vi "Excel Packing & Format.vi"(0 "Settings Cluster":T1={"Supply Voltage [Vdc]"=14.4, "Max Supply Current [Idc]"=50.0, "Settling Delay"=0.0, "Temp Criteria"=0.0, "Voltage Steps [Vrms]"=[0.0, 0.25, 0.5, 1.0, 1.95, 3.0, 3.9, 5.5], "User Notes"="", "Config Wave File Path"=path "", "Config Voltage [Vrms]"=0.1, "Channel Configuration List"={"Channel Configuration Cluster"={"Input"=enum."1 AVG", "Enable"=FALSE, "User Notes"="", "Voltage Range"=15.0, "Current Range"=2.5}, "Channel Configuration Cluster 2"={"Input"=enum."1", "Enable"=FALSE, "User Notes"="", "Voltage Range"=15.0, "Current Range"=2.5}, "Channel Configuration Cluster 3"={"Input"=enum."1", "Enable"=FALSE, "User Notes"="", "Voltage Range"=15.0, "Current Range"=2.5}, "Channel Configuration Cluster 4"={"Input"=enum."1", "Enable"=FALSE, "User Notes"="", "Voltage Range"=15.0, "Current Range"=2.5}, "Channel Configuration Cluster 5"={"Input"=enum."1", "Enable"=FALSE, "User Notes"="", "Voltage Range"=15.0, "Current Range"=2.5}, "Channel Configuration Cluster 6"={"Input"=enum."1", "Enable"=FALSE, "User Notes"="", "Voltage Range"=15.0, "Current Range"=2.5}, "Channel Configuration Cluster 7"={"Input"=enum."1", "Enable"=FALSE, "User Notes"="", "Voltage Range"=15.0, "Current Range"=2.5}, "Channel Configuration Cluster 8"={"Input"=enum."1", "Enable"=FALSE, "User Notes"="", "Voltage Range"=15.0, "Current Range"=2.5}, "Channel Configuration Cluster 9"={"Input"=enum."1", "Enable"=FALSE, "User Notes"="", "Voltage Range"=15.0, "Current Range"=2.5}, "Channel Configuration Cluster 10"={"Input"=enum."1", "Enable"=FALSE, "User Notes"="", "Voltage Range"=15.0, "Current Range"=25.0}, "Channel Configuration Cluster 11"={"Input"=enum."1", "Enable"=FALSE, "User Notes"="", "Voltage Range"=15.0, "Current Range"=25.0}, "Channel Configuration Cluster 12"={"Input"=enum."1", "Enable"=FALSE, "User Notes"="", "Voltage Range"=15.0, "Current Range"=25.0}, "Channel Configuration Cluster 13"={"Input"=enum."1", "Enable"=FALSE, "User Notes"="", "Voltage Range"=15.0, "Current Range"=25.0}, "Channel Configuration Cluster 14"={"Input"=enum."1", "Enable"=FALSE, "User Notes"="", "Voltage Range"=15.0, "Current Range"=25.0}, "Channel Configuration Cluster 15"={"Input"=enum."1", "Enable"=FALSE, "User Notes"="", "Voltage Range"=15.0, "Current Range"=25.0}, "Channel Configuration Cluster 16"={"Input"=enum."1", "Enable"=FALSE, "User Notes"="", "Voltage Range"=15.0, "Current Range"=25.0}, "Channel Configuration Cluster 17"={"Input"=enum."1", "Enable"=FALSE, "User Notes"="", "Voltage Range"=15.0, "Current Range"=25.0}}, "User Gains"={"Gain 1"=0.0, "Gain 2"=0.0, "Gain 3"=0.0, "Gain 4"=0.0, "Gain 5"=0.0, "Gain 6"=0.0}, "Gains"={"Gain 1"=0.0, "Gain 2"=0.0, "Gain 3"=0.0, "Gain 4"=0.0, "Gain 5"=0.0, "Gain 6"=0.0}, "Gain Array"={"Gain 1"=0.0, "Gain 2"=0.0, "Gain 3"=0.0, "Gain 4"=0.0, "Gain 5"=0.0, "Gain 6"=0.0, "Gain 7"=0.0, "Gain 8"=0.0, "Gain 9"=0.0, "Gain 10"=0.0, "Gain 11"=0.0, "Gain 12"=0.0, "Gain 13"=0.0, "Gain 14"=0.0, "Gain 15"=0.0, "Gain 16"=0.0, "Gain 17"=0.0}, "Wave File Path 1"=path "", "Wave File Path 2"=path "", "Wave File Path 3"=path "", "Wave File Path 4"=path "", "Range"=FALSE, "CF"=FALSE} {"Gain Array"."Gain 17" format="%.2f"; "Gain Array"."Gain 16" format="%.2f"; "Gain Array"."Gain 15" format="%.2f"; "Gain Array"."Gain 14" format="%.2f"; "Gain Array"."Gain 13" format="%.2f"; "Gain Array"."Gain 12" format="%.2f"; "Gain Array"."Gain 11" format="%.2f"; "Gain Array"."Gain 10" format="%.2f"; "Gain Array"."Gain 9" format="%.2f"; "Gain Array"."Gain 8" format="%.2f"; "Gain Array"."Gain 7" format="%.2f"; "Gain Array"."Gain 6" format="%.2f"; "Gain Array"."Gain 5" format="%.2f"; "Gain Array"."Gain 4" format="%.2f"; "Gain Array"."Gain 3" format="%.2f"; "Gain Array"."Gain 2" format="%.2f"; "Gain Array"."Gain 1" format="%.2f"; "Gains"."Gain 6" format="%.2f"; "Gains"."Gain 5" format="%.2f"; "Gains"."Gain 4" format="%.2f"; "Gains"."Gain 3" format="%.2f"; "Gains"."Gain 2" format="%.2f"; "Gains"."Gain 1" format="%.2f"; "User Gains"."Gain 6" format="%.2f"; "User Gains"."Gain 5" format="%.2f"; "User Gains"."Gain 4" format="%.2f"; "User Gains"."Gain 3" format="%.2f"; "User Gains"."Gain 2" format="%.2f"; "User Gains"."Gain 1" format="%.2f"; "Channel Configuration List"."Channel Configuration Cluster 17"."Current Range" items=["1 <500m>"=0.5, "2 <1>"=1.0, "5 <2.5>"=2.5, "10 <5>"=5.0, "20 <10>"=10.0, "50 <25>"=25.0]; "Channel Configuration List"."Channel Configuration Cluster 17"."Voltage Range" items=["1.5 <0.75>"=0.75, "3 <1.5>"=1.5, "6 <3>"=3.0, "10 <5>"=5.0, "15 <7.5>"=7.5, "30 <15>"=15.0, "60 <30>"=30.0, "100 <50>"=50.0, "150 <75>"=75.0, "300 <150>"=150.0, "600 <300>"=300.0, "1000 <500>"=500.0]; "Channel Configuration List"."Channel Configuration Cluster 16"."Current Range" items=["1 <500m>"=0.5, "2 <1>"=1.0, "5 <2.5>"=2.5, "10 <5>"=5.0, "20 <10>"=10.0, "50 <25>"=25.0]; "Channel Configuration List"."Channel Configuration Cluster 16"."Voltage Range" items=["1.5 <0.75>"=0.75, "3 <1.5>"=1.5, "6 <3>"=3.0, "10 <5>"=5.0, "15 <7.5>"=7.5, "30 <15>"=15.0, "60 <30>"=30.0, "100 <50>"=50.0, "150 <75>"=75.0, "300 <150>"=150.0, "600 <300>"=300.0, "1000 <500>"=500.0]; "Channel Configuration List"."Channel Configuration Cluster 15"."Current Range" items=["1 <500m>"=0.5, "2 <1>"=1.0, "5 <2.5>"=2.5, "10 <5>"=5.0, "20 <10>"=10.0, "50 <25>"=25.0]; "Channel Configuration List"."Channel Configuration Cluster 15"."Voltage Range" items=["1.5 <0.75>"=0.75, "3 <1.5>"=1.5, "6 <3>"=3.0, "10 <5>"=5.0, "15 <7.5>"=7.5, "30 <15>"=15.0, "60 <30>"=30.0, "100 <50>"=50.0, "150 <75>"=75.0, "300 <150>"=150.0, "600 <300>"=300.0, "1000 <500>"=500.0]; "Channel Configuration List"."Channel Configuration Cluster 14"."Current Range" items=["1 <500m>"=0.5, "2 <1>"=1.0, "5 <2.5>"=2.5, "10 <5>"=5.0, "20 <10>"=10.0, "50 <25>"=25.0]; "Channel Configuration List"."Channel Configuration Cluster 14"."Voltage Range" items=["1.5 <0.75>"=0.75, "3 <1.5>"=1.5, "6 <3>"=3.0, "10 <5>"=5.0, "15 <7.5>"=7.5, "30 <15>"=15.0, "60 <30>"=30.0, "100 <50>"=50.0, "150 <75>"=75.0, "300 <150>"=150.0, "600 <300>"=300.0, "1000 <500>"=500.0]; "Channel Configuration List"."Channel Configuration Cluster 13"."Current Range" items=["1 <500m>"=0.5, "2 <1>"=1.0, "5 <2.5>"=2.5, "10 <5>"=5.0, "20 <10>"=10.0, "50 <25>"=25.0]; "Channel Configuration List"."Channel Configuration Cluster 13"."Voltage Range" items=["1.5 <0.75>"=0.75, "3 <1.5>"=1.5, "6 <3>"=3.0, "10 <5>"=5.0, "15 <7.5>"=7.5, "30 <15>"=15.0, "60 <30>"=30.0, "100 <50>"=50.0, "150 <75>"=75.0, "300 <150>"=150.0, "600 <300>"=300.0, "1000 <500>"=500.0]; "Channel Configuration List"."Channel Configuration Cluster 12"."Current Range" items=["1 <500m>"=0.5, "2 <1>"=1.0, "5 <2.5>"=2.5, "10 <5>"=5.0, "20 <10>"=10.0, "50 <25>"=25.0]; "Channel Configuration List"."Channel Configuration Cluster 12"."Voltage Range" items=["1.5 <0.75>"=0.75, "3 <1.5>"=1.5, "6 <3>"=3.0, "10 <5>"=5.0, "15 <7.5>"=7.5, "30 <15>"=15.0, "60 <30>"=30.0, "100 <50>"=50.0, "150 <75>"=75.0, "300 <150>"=150.0, "600 <300>"=300.0, "1000 <500>"=500.0]; "Channel Configuration List"."Channel Configuration Cluster 11"."Current Range" items=["1 <500m>"=0.5, "2 <1>"=1.0, "5 <2.5>"=2.5, "10 <5>"=5.0, "20 <10>"=10.0, "50 <25>"=25.0]; "Channel Configuration List"."Channel Configuration Cluster 11"."Voltage Range" items=["1.5 <0.75>"=0.75, "3 <1.5>"=1.5, "6 <3>"=3.0, "10 <5>"=5.0, "15 <7.5>"=7.5, "30 <15>"=15.0, "60 <30>"=30.0, "100 <50>"=50.0, "150 <75>"=75.0, "300 <150>"=150.0, "600 <300>"=300.0, "1000 <500>"=500.0]; "Channel Configuration List"."Channel Configuration Cluster 10"."Current Range" items=["1 <500m>"=0.5, "2 <1>"=1.0, "5 <2.5>"=2.5, "10 <5>"=5.0, "20 <10>"=10.0, "50 <25>"=25.0]; "Channel Configuration List"."Channel Configuration Cluster 10"."Voltage Range" items=["1.5 <0.75>"=0.75, "3 <1.5>"=1.5, "6 <3>"=3.0, "10 <5>"=5.0, "15 <7.5>"=7.5, "30 <15>"=15.0, "60 <30>"=30.0, "100 <50>"=50.0, "150 <75>"=75.0, "300 <150>"=150.0, "600 <300>"=300.0, "1000 <500>"=500.0]; "Channel Configuration List"."Channel Configuration Cluster 9"."Voltage Range" items=["1.5 <0.75>"=0.75, "3 <1.5>"=1.5, "6 <3>"=3.0, "10 <5>"=5.0, "15 <7.5>"=7.5, "30 <15>"=15.0, "60 <30>"=30.0, "100 <50>"=50.0, "150 <75>"=75.0, "300 <150>"=150.0, "600 <300>"=300.0, "1000 <500>"=500.0]; "Channel Configuration List"."Channel Configuration Cluster 9"."Current Range" items=["10m <5m>"=0.005, "20m <10m>"=0.01, "50m <25m>"=0.025, "100m <50m>"=0.05, "200m <100m>"=0.1, "500m <250m>"=0.25, "1 <500m>"=0.5, "2 <1>"=1.0, "5 <2.5>"=2.5]; "Channel Configuration List"."Channel Configuration Cluster 8"."Voltage Range" items=["1.5 <0.75>"=0.75, "3 <1.5>"=1.5, "6 <3>"=3.0, "10 <5>"=5.0, "15 <7.5>"=7.5, "30 <15>"=15.0, "60 <30>"=30.0, "100 <50>"=50.0, "150 <75>"=75.0, "300 <150>"=150.0, "600 <300>"=300.0, "1000 <500>"=500.0]; "Channel Configuration List"."Channel Configuration Cluster 8"."Current Range" items=["10m <5m>"=0.005, "20m <10m>"=0.01, "50m <25m>"=0.025, "100m <50m>"=0.05, "200m <100m>"=0.1, "500m <250m>"=0.25, "1 <500m>"=0.5, "2 <1>"=1.0, "5 <2.5>"=2.5]; "Channel Configuration List"."Channel Configuration Cluster 7"."Voltage Range" items=["1.5 <0.75>"=0.75, "3 <1.5>"=1.5, "6 <3>"=3.0, "10 <5>"=5.0, "15 <7.5>"=7.5, "30 <15>"=15.0, "60 <30>"=30.0, "100 <50>"=50.0, "150 <75>"=75.0, "300 <150>"=150.0, "600 <300>"=300.0, "1000 <500>"=500.0]; "Channel Configuration List"."Channel Configuration Cluster 7"."Current Range" items=["10m <5m>"=0.005, "20m <10m>"=0.01, "50m <25m>"=0.025, "100m <50m>"=0.05, "200m <100m>"=0.1, "500m <250m>"=0.25, "1 <500m>"=0.5, "2 <1>"=1.0, "5 <2.5>"=2.5]; "Channel Configuration List"."Channel Configuration Cluster 6"."Voltage Range" items=["1.5 <0.75>"=0.75, "3 <1.5>"=1.5, "6 <3>"=3.0, "10 <5>"=5.0, "15 <7.5>"=7.5, "30 <15>"=15.0, "60 <30>"=30.0, "100 <50>"=50.0, "150 <75>"=75.0, "300 <150>"=150.0, "600 <300>"=300.0, "1000 <500>"=500.0]; "Channel Configuration List"."Channel Configuration Cluster 6"."Current Range" items=["10m <5m>"=0.005, "20m <10m>"=0.01, "50m <25m>"=0.025, "100m <50m>"=0.05, "200m <100m>"=0.1, "500m <250m>"=0.25, "1 <500m>"=0.5, "2 <1>"=1.0, "5 <2.5>"=2.5]; "Channel Configuration List"."Channel Configuration Cluster 5"."Voltage Range" items=["1.5 <0.75>"=0.75, "3 <1.5>"=1.5, "6 <3>"=3.0, "10 <5>"=5.0, "15 <7.5>"=7.5, "30 <15>"=15.0, "60 <30>"=30.0, "100 <50>"=50.0, "150 <75>"=75.0, "300 <150>"=150.0, "600 <300>"=300.0, "1000 <500>"=500.0]; "Channel Configuration List"."Channel Configuration Cluster 5"."Current Range" items=["10m <5m>"=0.005, "20m <10m>"=0.01, "50m <25m>"=0.025, "100m <50m>"=0.05, "200m <100m>"=0.1, "500m <250m>"=0.25, "1 <500m>"=0.5, "2 <1>"=1.0, "5 <2.5>"=2.5]; "Channel Configuration List"."Channel Configuration Cluster 4"."Voltage Range" items=["1.5 <0.75>"=0.75, "3 <1.5>"=1.5, "6 <3>"=3.0, "10 <5>"=5.0, "15 <7.5>"=7.5, "30 <15>"=15.0, "60 <30>"=30.0, "100 <50>"=50.0, "150 <75>"=75.0, "300 <150>"=150.0, "600 <300>"=300.0, "1000 <500>"=500.0]; "Channel Configuration List"."Channel Configuration Cluster 4"."Current Range" items=["10m <5m>"=0.005, "20m <10m>"=0.01, "50m <25m>"=0.025, "100m <50m>"=0.05, "200m <100m>"=0.1, "500m <250m>"=0.25, "1 <500m>"=0.5, "2 <1>"=1.0, "5 <2.5>"=2.5]; "Channel Configuration List"."Channel Configuration Cluster 3"."Voltage Range" items=["1.5 <0.75>"=0.75, "3 <1.5>"=1.5, "6 <3>"=3.0, "10 <5>"=5.0, "15 <7.5>"=7.5, "30 <15>"=15.0, "60 <30>"=30.0, "100 <50>"=50.0, "150 <75>"=75.0, "300 <150>"=150.0, "600 <300>"=300.0, "1000 <500>"=500.0]; "Channel Configuration List"."Channel Configuration Cluster 3"."Current Range" items=["10m <5m>"=0.005, "20m <10m>"=0.01, "50m <25m>"=0.025, "100m <50m>"=0.05, "200m <100m>"=0.1, "500m <250m>"=0.25, "1 <500m>"=0.5, "2 <1>"=1.0, "5 <2.5>"=2.5]; "Channel Configuration List"."Channel Configuration Cluster 2"."Voltage Range" items=["1.5 <0.75>"=0.75, "3 <1.5>"=1.5, "6 <3>"=3.0, "10 <5>"=5.0, "15 <7.5>"=7.5, "30 <15>"=15.0, "60 <30>"=30.0, "100 <50>"=50.0, "150 <75>"=75.0, "300 <150>"=150.0, "600 <300>"=300.0, "1000 <500>"=500.0]; "Channel Configuration List"."Channel Configuration Cluster 2"."Current Range" items=["10m <5m>"=0.005, "20m <10m>"=0.01, "50m <25m>"=0.025, "100m <50m>"=0.05, "200m <100m>"=0.1, "500m <250m>"=0.25, "1 <500m>"=0.5, "2 <1>"=1.0, "5 <2.5>"=2.5]; "Channel Configuration List"."Channel Configuration Cluster"."Voltage Range" items=["1.5 <0.75>"=0.75, "3 <1.5>"=1.5, "6 <3>"=3.0, "10 <5>"=5.0, "15 <7.5>"=7.5, "30 <15>"=15.0, "60 <30>"=30.0, "100 <50>"=50.0, "150 <75>"=75.0, "300 <150>"=150.0, "600 <300>"=300.0, "1000 <500>"=500.0]; "Channel Configuration List"."Channel Configuration Cluster"."Current Range" items=["10m <5m>"=0.005, "20m <10m>"=0.01, "50m <25m>"=0.025, "100m <50m>"=0.05, "200m <100m>"=0.1, "500m <250m>"=0.25, "1 <500m>"=0.5, "2 <1>"=1.0, "5 <2.5>"=2.5]; "Settling Delay" min=0.0 format="%<%H:%M:%S>t"}, 1 "Datalog Cluster Array":T7[](array[typedef]) {"WT1800 Averages"."Vrms" format="%.3f"; "WT1800 Averages"."Irms" format="%.3f"; "WT1800 Averages"."Power" format="%.3f"; "WT1800 Averages"."Vpkpk" format="%.3f"; "WT1800 Averages"."Ipkpk" format="%.3f"; "WT1800 Measurements"."Vrms" format="%.3f"; "WT1800 Measurements"."Irms" format="%.3f"; "WT1800 Measurements"."Power" format="%.3f"; "WT1800 Measurements"."Vpkpk" format="%.3f"; "WT1800 Measurements"."Ipkpk" format="%.3f"; "DSA Averages"."Vrms" format="%.3f"; "DSA Averages"."Vdc" format="%.3f"; "DSA Averages"."Vpk+" format="%.3f"; "DSA Averages"."Vpk-" format="%.3f"; "DSA Averages"."Vpkpk" format="%.3f"; "DSA Measurements"."Vrms" format="%.3f"; "DSA Measurements"."Vdc" format="%.3f"; "DSA Measurements"."Vpk+" format="%.3f"; "DSA Measurements"."Vpk-" format="%.3f"; "DSA Measurements"."Vpkpk" format="%.3f"}) -> (7 "Irms":dbl[][](array[numeric]), 8 "Heat":dbl[](array[numeric]), 9 "Power":dbl[][](array[numeric]), 10 "DSA Averages":T13[][](array[typedef]) {"Vrms" format="%.3f"; "Vdc" format="%.3f"; "Vpk+" format="%.3f"; "Vpk-" format="%.3f"; "Vpkpk" format="%.3f"}, 11 "Vrms":dbl[][](array[numeric]), 12 "Enable CH":bool[](array[boolean]), 13 "Vpp":dbl[][](array[numeric]), 14 "Voltage Steps [Vrms]":dbl[](array[numeric]), 15 "Voltage Step":string[](array[string]), 16 "CH#":string[](array[string]), 17 "Ipp":dbl[][](array[numeric]), 18 "WT1800 Averages":T10[][](array[typedef]) {"Vrms" format="%.3f"; "Irms" format="%.3f"; "Power" format="%.3f"; "Vpkpk" format="%.3f"; "Ipkpk" format="%.3f"}, 19 "Cluster":T14)   [LabVIEW 2015]
uses:
  Controls/DSA Readings.ctl
  Controls/WT1800 Readings.ctl
  Controls/Datalog Bundle Control.ctl
  Controls/WT1800 Functions.ctl
  Controls/WT1800 Measurements.ctl
  Controls/DSA Functions.ctl
  Controls/DSA Measurements.ctl
  Controls/Settings Control.ctl
  Controls/Channel Configuration List.ctl
  Controls/Channel Configuration Cluster.ctl
  Controls/Channel Configuration Cluster High Current.ctl
  Controls/Gain Averages.ctl
  Controls/Gain Array.ctl
panel:
  out "NICH1_Vrms":string[](array[string])
  out "NICH2_Vrms":string[](array[string])
  out "NICH2_Vpp":string[](array[string])
  out "NICH1_Vpp":string[](array[string])
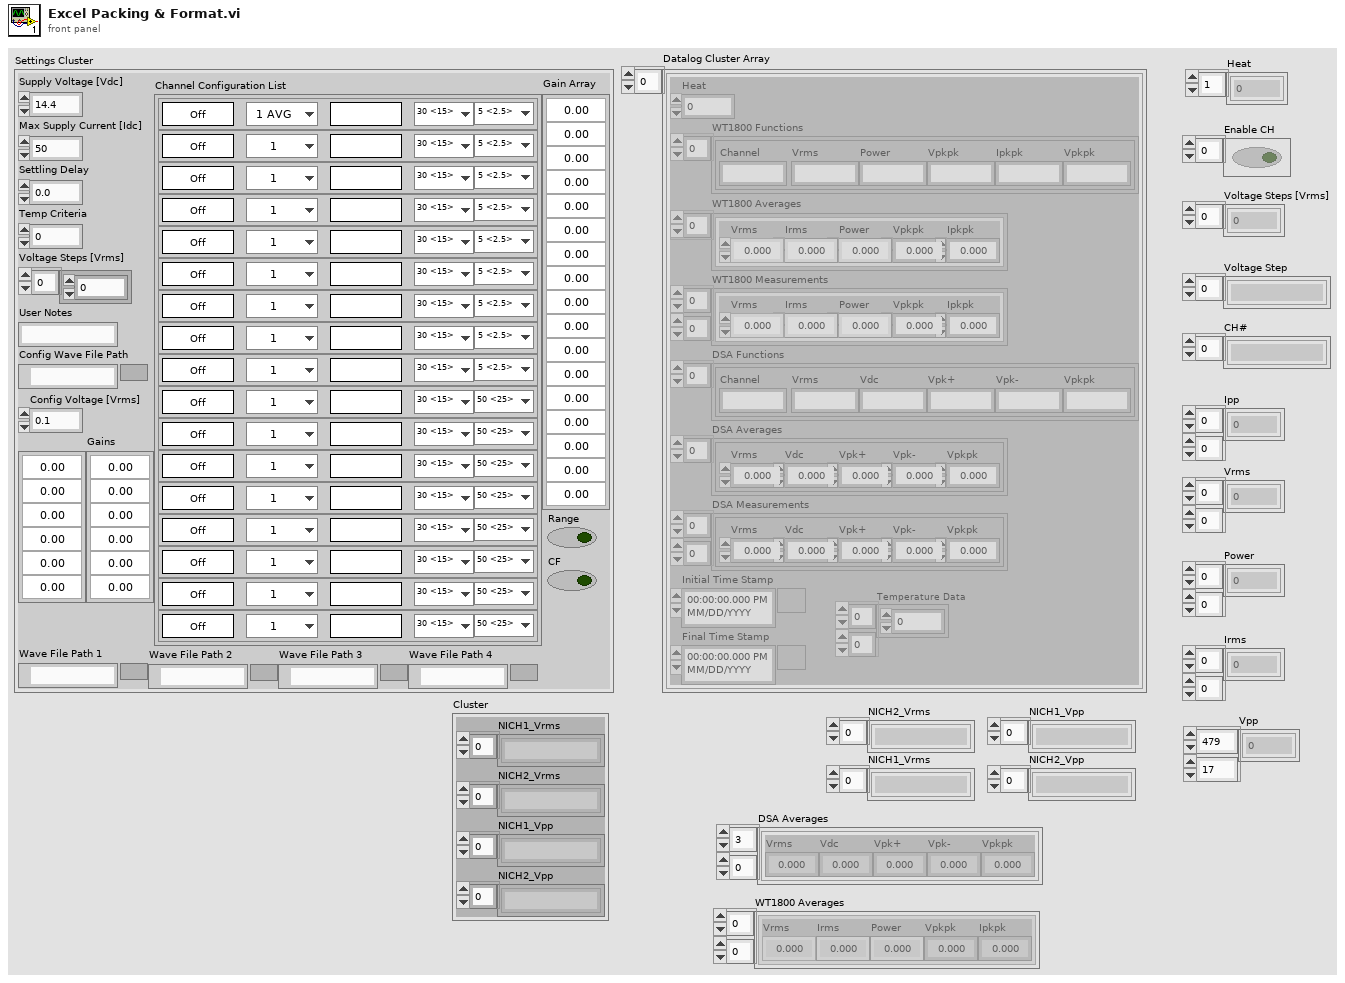
[diagram p1: front panel]
types:
  T1 = typedef "Settings Control.ctl" = cluster{"Supply Voltage [Vdc]":dbl, "Max Supply Current [Idc]":dbl, "Settling Delay":dbl, "Temp Criteria":dbl, "Voltage Steps [Vrms]":dbl[], "User Notes":string, "Config Wave File Path":path, "Config Voltage [Vrms]":dbl, "Channel Configuration List":T2, "User Gains":T5, "Gains":T5, "Gain Array":T6, "Wave File Path 1":path, "Wave File Path 2":path, "Wave File Path 3":path, "Wave File Path 4":path, "Range":bool, "CF":bool}
  T2 = typedef "Channel Configuration List.ctl" = cluster{"Channel Configuration Cluster":T3, "Channel Configuration Cluster 2":T3, "Channel Configuration Cluster 3":T3, "Channel Configuration Cluster 4":T3, "Channel Configuration Cluster 5":T3, "Channel Configuration Cluster 6":T3, "Channel Configuration Cluster 7":T3, "Channel Configuration Cluster 8":T3, "Channel Configuration Cluster 9":T3, "Channel Configuration Cluster 10":T4, "Channel Configuration Cluster 11":T4, "Channel Configuration Cluster 12":T4, "Channel Configuration Cluster 13":T4, "Channel Configuration Cluster 14":T4, "Channel Configuration Cluster 15":T4, "Channel Configuration Cluster 16":T4, "Channel Configuration Cluster 17":T4}
  T3 = typedef "Channel Configuration Cluster.ctl" = cluster{"Input":enum16{"---", "1", "1 AVG", "2", "2 AVG", "3", "3 AVG", "4", "4 AVG"}, "Enable":bool, "User Notes":string, "Voltage Range":dbl, "Current Range":dbl}
  T4 = typedef "Channel Configuration Cluster High Current.ctl" = cluster{"Input":enum16{"---", "1", "1 AVG", "2", "2 AVG", "3", "3 AVG", "4", "4 AVG"}, "Enable":bool, "User Notes":string, "Voltage Range":dbl, "Current Range":dbl}
  T5 = typedef "Gain Averages.ctl" = cluster{"Gain 1":dbl, "Gain 2":dbl, "Gain 3":dbl, "Gain 4":dbl, "Gain 5":dbl, "Gain 6":dbl}
  T6 = typedef "Gain Array.ctl" = cluster{"Gain 1":dbl, "Gain 2":dbl, "Gain 3":dbl, "Gain 4":dbl, "Gain 5":dbl, "Gain 6":dbl, "Gain 7":dbl, "Gain 8":dbl, "Gain 9":dbl, "Gain 10":dbl, "Gain 11":dbl, "Gain 12":dbl, "Gain 13":dbl, "Gain 14":dbl, "Gain 15":dbl, "Gain 16":dbl, "Gain 17":dbl}
  T7 = typedef "Datalog Bundle Control.ctl" = cluster{"Heat":dbl, "WT1800 Functions":T8, "WT1800 Averages":T9, "WT1800 Measurements":T10[][], "DSA Functions":T11, "DSA Averages":T12, "DSA Measurements":T13[][], "Initial Time Stamp":timestamp, "Final Time Stamp":timestamp, "Temperature Data":dbl[][]}
  T8 = typedef "WT1800 Functions.ctl" = cluster{"Channel":string, "Vrms":string, "Power":string, "Vpkpk":string, "Ipkpk":string, "Vpkpk":string}[]
  T9 = typedef "WT1800 Measurements.ctl" = T10[]
  T10 = typedef "WT1800 Readings.ctl" = cluster{"Vrms":dbl, "Irms":dbl, "Power":dbl, "Vpkpk":dbl, "Ipkpk":dbl}
  T11 = typedef "DSA Functions.ctl" = cluster{"Channel":string, "Vrms":string, "Vdc":string, "Vpk+":string, "Vpk-":string, "Vpkpk":string}[]
  T12 = typedef "DSA Measurements.ctl" = T13[]
  T13 = typedef "DSA Readings.ctl" = cluster{"Vrms":dbl, "Vdc":dbl, "Vpk+":dbl, "Vpk-":dbl, "Vpkpk":dbl}
  T14 = cluster{"NICH1_Vrms":string[], "NICH2_Vrms":string[], "NICH1_Vpp":string[], "NICH2_Vpp":string[]}
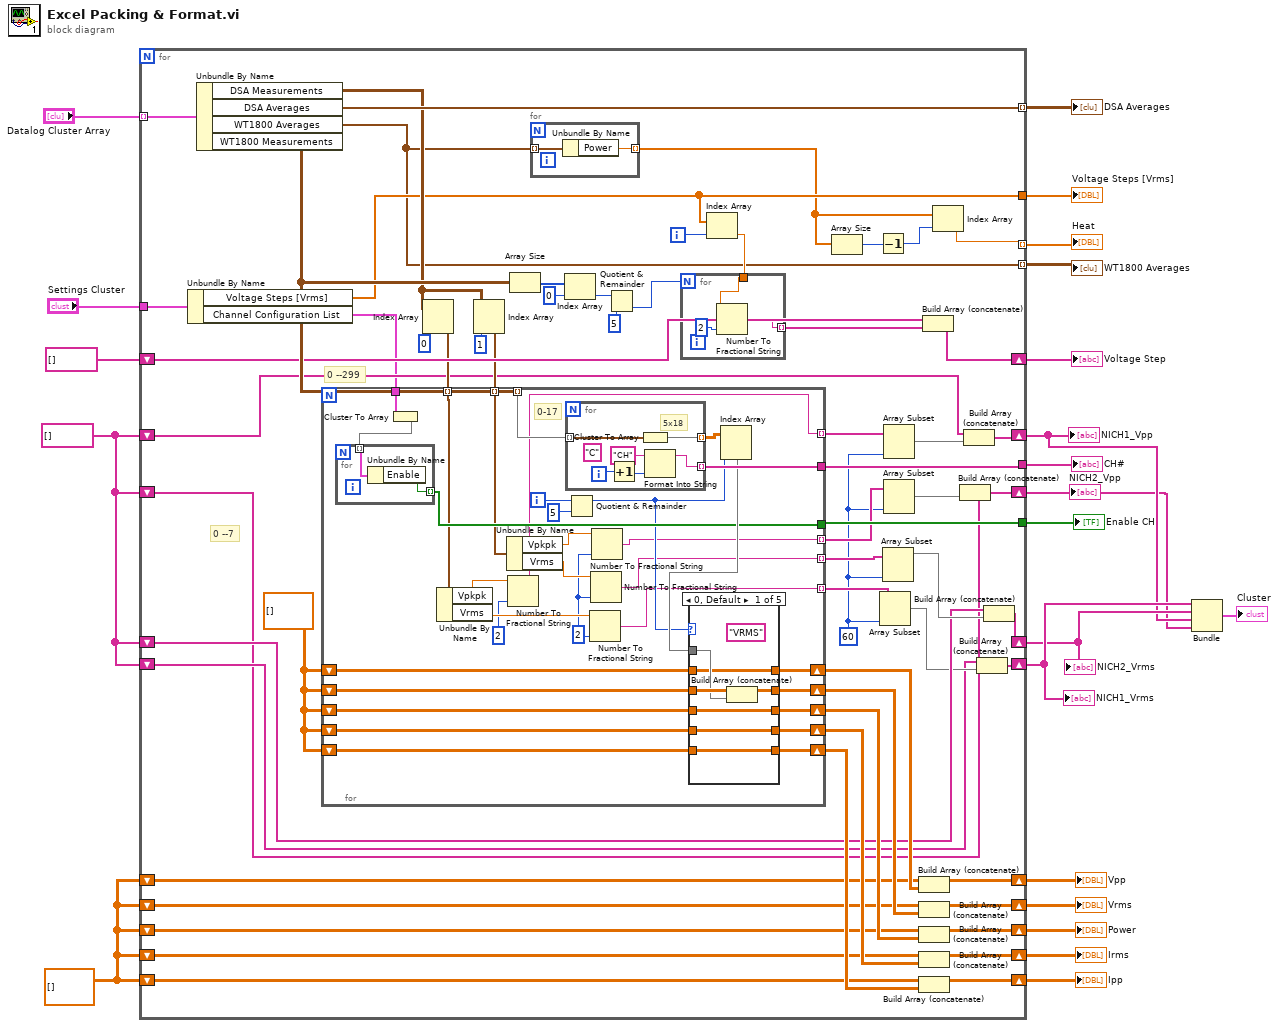
[diagram p0: block diagram]
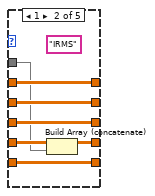
[diagram p2: hidden frame]
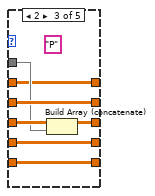
[diagram p3: hidden frame]
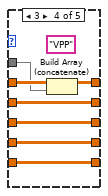
[diagram p4: hidden frame]
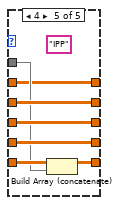
[diagram p5: hidden frame]
diagram:
  w8 = string[] []
  w9 = dbl[][] []
  n1 = for {
    tunnel: [w73] -> w16
    tunnel: [w24] -> w17 mode=indexing
    tunnel: [w26] -> w18
    tunnel: [w71] -> w22 mode=indexing
    tunnel: [w65] -> w20
    tunnel: [w63] -> w21 mode=indexing
    shift-right: [w61] -> w11
    shift-left: w9 -> [w62]
    shift-right: [w59] -> w12
    shift-left: w9 -> [w60]
    shift-right: [w57] -> w13
    shift-left: w9 -> [w58]
    shift-right: [w55] -> w14
    shift-left: w9 -> [w56]
    shift-right: [w53] -> w15
    shift-left: w9 -> [w54]
    shift-right: [w51] -> w19
    shift-left: string[] [] -> [w52]
    shift-right: [w40] -> w7
    shift-left: w8 -> [w38]
    shift-right: [w41] -> w6
    shift-left: w8 -> [w42]
    shift-right: [w31] -> w5
    shift-left: w8 -> [w30]
    shift-right: [w37] -> w4
    shift-left: w8 -> [w36]
    tunnel: "Datalog Cluster Array" -> [w28] mode=indexing
    tunnel: "Settings Cluster" -> [w27]
    i -> [w69]
    w34 = 60 ("length")
    w64 = dbl[][] []
    # "0 --299"
    # "0 --7"
    n2 = Unbundle By Name(w27) -> ("Voltage Steps [Vrms]"=w26:dbl[], "Channel Configuration List"=w25:T2)
    n3 = Unbundle By Name(w28) -> ("DSA Measurements"=w46:T13[][], "DSA Averages"=w63:T12, "WT1800 Averages"=w24:T9, "WT1800 Measurements"=w83:T10[][])
    n4 = Index Array(array=w46, index (col)=0 ("disabled index (col)")) -> (element=w50:T13[])  [unwired: 1 in]
    n5 = Index Array(array=w46, index (col)=1 ("disabled index (col)")) -> (element=w47:T13[])  [unwired: 1 in]
    n6 = for {
      tunnel: w83 -> [w120] mode=indexing
      tunnel: [w118] -> w73
      shift-right: [w114] -> w75
      shift-left: w64 -> [w113]
      shift-right: [w112] -> w77
      shift-left: w64 -> [w111]
      shift-right: [w110] -> w74
      shift-left: w64 -> [w109]
      shift-right: [w107] -> w76
      shift-left: w64 -> [w108]
      shift-right: [w105] -> w78
      shift-left: w64 -> [w106]
      tunnel: w25 -> [w104]
      tunnel: [w102] -> w65
      tunnel: w50 -> [w100] mode=indexing
      tunnel: w47 -> [w99] mode=indexing
      tunnel: [w95] -> w45 mode=indexing
      tunnel: [w97] -> w44 mode=indexing
      tunnel: [w89] -> w35 mode=indexing
      tunnel: [w92] -> w33 mode=indexing
      i -> [w117]
      w90 = i16 2 ("width (-)")
      # "0-17"
      n7 = Cluster To Array(cluster=w104) -> (array=w103:T4[])
      n8 = for {
        tunnel: w103 -> [w122] mode=indexing
        tunnel: [w121] -> w102 mode=indexing
        n9 = Unbundle By Name(w122) -> ("Enable"=w121:bool)
      }
      n10 = Unbundle By Name(w100) -> ("Vpkpk"=w93:dbl, "Vrms"=w98:dbl)
      n11 = Unbundle By Name(w99) -> ("Vpkpk"=w91:dbl, "Vrms"=w96:dbl)
      n12 = Number To Fractional String(number=w93, precision (6)=i16 2 ("width (-)")) -> (F-format string=w92:string)  [unwired: 2 in]
      n13 = for {
        tunnel: w120 -> [w163] mode=indexing
        tunnel: [w162] -> w119 mode=indexing
        tunnel: [w159] -> w118 mode=indexing
        i -> [w160]
        (unwired) "C"
        # "5x18"
        n14 = Increment(x=w160) -> (x+1=w158:i32)
        n15 = Cluster To Array(cluster=w163) -> (array=w162:dbl[])
        n16 = Format Into String(initial string="CH", w158) -> (resulting string=w159:string)  [unwired: 2 in, 1 out]
      }
      n17 = Quotient & Remainder(x=w117, y=5) -> (x-y*floor(x/y)=w101:i32)  [unwired: 1 out]
      n18 = Number To Fractional String(number=w98, precision (6)=w90) -> (F-format string=w97:string)  [unwired: 2 in]
      n19 = Number To Fractional String(number=w96, precision (6)=w90) -> (F-format string=w95:string)  [unwired: 2 in]
      n20 = Number To Fractional String(number=w91, precision (6)=w90) -> (F-format string=w89:string)  [unwired: 2 in]
      n21 = Index Array(array=w119, index (col)=w101) -> (element=w115:dbl[])  [unwired: 1 in]
      n22 = case shown="0, Default" w101 {
        tunnel: w115 -> [w127 w131 w140 w146 w152]
        tunnel: [w128 w136 w143 w150 w157] -> w114
        tunnel: w113 -> [w129 w136 w143 w150 w157]
        tunnel: [w126 w135 w142 w149 w156] -> w112
        tunnel: w111 -> [w126 w135 w141 w149 w156]
        tunnel: [w124 w133 w138 w145 w155] -> w110
        tunnel: w109 -> [w124 w132 w138 w145 w155]
        tunnel: w108 -> [w123 w130 w137 w144 w153]
        tunnel: [w123 w130 w137 w144 w154] -> w107
        tunnel: w106 -> [w125 w134 w139 w147 w151]
        tunnel: [w125 w134 w139 w148 w151] -> w105
        frame 0, Default {
          (unwired) "VRMS" ("initial string")
          n23 = Build Array (concatenate)(w129, w127) -> (w128:dbl[][])
        }
        frame 1 {
          (unwired) "IRMS" ("initial string")
          n24 = Build Array (concatenate)(w132, w131) -> (w133:dbl[][])
        }
        frame 2 {
          (unwired) "P" ("initial string")
          n25 = Build Array (concatenate)(w141, w140) -> (w142:dbl[][])
        }
        frame 3 {
          (unwired) "VPP" ("initial string")
          n26 = Build Array (concatenate)(w147, w146) -> (w148:dbl[][])
        }
        frame 4 {
          (unwired) "IPP" ("initial string")
          n27 = Build Array (concatenate)(w153, w152) -> (w154:dbl[][])
        }
      }
    }
    n28 = Array Size(array=w83) -> (size(s)=w82:i32[])
    n29 = for {
      tunnel: [w84] -> w23 mode=indexing
      tunnel: w24 -> [w85] mode=indexing
      n30 = Unbundle By Name(w85) -> ("Power"=w84:dbl)
    }
    n31 = Index Array(array=w82, index=0) -> (element=w80:i32)
    n32 = Quotient & Remainder(x=w80, y=5) -> (floor(x/y)=w68:i32)  [unwired: 1 out]
    n33 = Index Array(array=w26, index=w69) -> (element=w67:dbl)
    n34 = for {
      N: w68 -> [_]
      tunnel: w67 -> [w88]
      tunnel: [w86] -> w66 mode=indexing
      n35 = Number To Fractional String(number=w88, precision (6)=i16 2 ("width (-)")) -> (F-format string=w86:string)  [unwired: 2 in]
    }
    n36 = Array Size(array=w23) -> (size(s)=w72:i32)
    n37 = Decrement(x=w72) -> (x-1=w70:i32)
    n38 = Array Subset(array=w44, length=w34) -> (w39:string[])  [unwired: 1 in]
    n39 = Array Subset(array=w45, length=w34) -> (w43:string[])  [unwired: 1 in]
    n40 = Array Subset(array=w33, length=w34) -> (w32:string[])  [unwired: 1 in]
    n41 = Array Subset(array=w35, length=w34) -> (w29:string[])  [unwired: 1 in]
    n42 = Build Array (concatenate)(w62, w78) -> (w61:dbl[][])
    n43 = Build Array (concatenate)(w56, w75) -> (w55:dbl[][])
    n44 = Build Array (concatenate)(w60, w77) -> (w59:dbl[][])
    n45 = Build Array (concatenate)(w54, w74) -> (w53:dbl[][])
    n46 = Build Array (concatenate)(w58, w76) -> (w57:dbl[][])
    n47 = Build Array (concatenate)(w52, w66) -> (w51:string[])
    n48 = Index Array(array=w23, index=w70) -> (element=w71:dbl)
    n49 = Build Array (concatenate)(w36, w29) -> (w37:string[])
    n50 = Build Array (concatenate)(w30, w32) -> (w31:string[])
    n51 = Build Array (concatenate)(w38, w39) -> (w40:string[])
    n52 = Build Array (concatenate)(w42, w43) -> (w41:string[])
  }
  "Heat" <- w22
  "DSA Averages" <- w21
  "Enable CH" <- w20
  "Voltage Step" <- w19
  "Voltage Steps [Vrms]" <- w18
  "WT1800 Averages" <- w17
  "CH#" <- w16
  "Irms" <- w15
  "Vrms" <- w14
  "Ipp" <- w13
  "Power" <- w12
  "Vpp" <- w11
  "NICH1_Vpp" <- w5
  "NICH2_Vpp" <- w4
  "NICH2_Vrms" <- w6
  "NICH1_Vrms" <- w7
  n53 = Bundle(w7, w6, w5, w4) -> (→"Cluster":cluster{string[], string[], string[], string[]})  [unwired: 1 in]
